vi "Get DDG External Output Enabled.vi"(10 "puiEnabled":u32, 11 "uiIndex":u32) -> (2 "puiEnabled out":u32, 3 "function return":u32)   [LabVIEW 2018, in "AndorSDK.lvlib"]
doc: "EXPNETTYPE unsigned int WINAPI GetDDGExternalOutputEnabled(at_u32 uiIndex, at_u32 * puiEnabled);"
uses:
  AndorSDK.lvlib
  ATMCD32D.dll
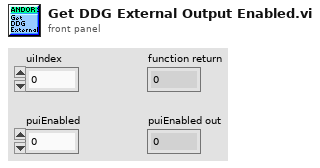
[diagram p1: front panel]
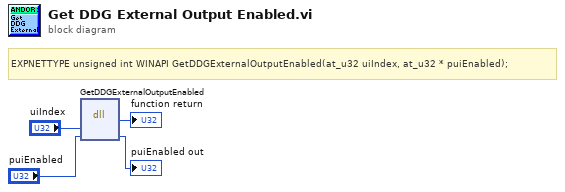
[diagram p0: block diagram]
diagram:
  # "EXPNETTYPE unsigned int WINAPI GetDDGExternalOutputEnabled(at_u32 uiIndex, at_u32 * puiEnabled);"
  n1 = dll-call lib="PTH2babs E\nPersönliches02 - Arbeit03-HiwijobsLabviewCodelibANDOR\tAndor SDK\nATMCD32D.*" fn="GetDDGExternalOutputEnabled"("uiIndex"="uiIndex", "puiEnabled"="puiEnabled") -> (→"function return":u32, "puiEnabled"=→"puiEnabled out":u32)  [unwired: 4 in, 2 out]
